vi "Match.vi"(10 "log record":T1 {"timestamp" format="%<%x %.3X>T"}, 11 "regex":refnum<class "Regex.lvclass">) -> (2 "matches":bool[](array[boolean]), 3 "dup regex":refnum<class "Regex.lvclass">)   [LabVIEW 2018, in "Logging.lvlib" / "Regex.lvclass"]
uses:
  Regex.lvclass
  Log Record.ctl
  Logger/Internal Log Levels.ctl
  Regex.lvclass/Regex.ctl
  <vilib>/regexp/Match Regular Expression.xnode
  Logging.lvlib
panel:
  # "Connector Pane"
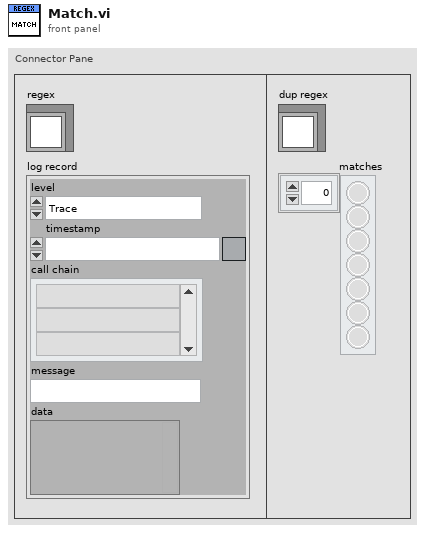
[diagram p1: front panel]
types:
  T1 = typedef "Logging.lvlib/Log Record.ctl" = cluster{"level":T2, "timestamp":timestamp, "call chain":string[], "message":string, "data":variant}
  T2 = typedef "Logging.lvlib/Internal Log Levels.ctl" = enum16{"Trace", "Debug", "Info", "Warning", "Error", "Critical", "Internal"}
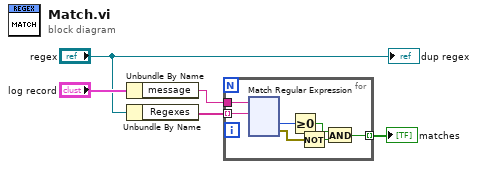
[diagram p0: block diagram]
diagram:
  n1 = Unbundle By Name("log record") -> ("message"=w4:string)
  n2 = Unbundle By Name("regex") -> ("Regexes"=w3:string[])
  n3 = for {
    tunnel: w4 -> [w12]
    tunnel: w3 -> [w11] mode=indexing
    tunnel: [w7] -> w1 mode=indexing
    n4 = xnode "Match Regular Expression"("input string"=w12, "regular expression"=w11) -> ("offset past match"=w10:i32, "error out"=w8:errorcluster)  [unwired: 4 in, 3 out]
    n5 = Greater Or Equal To 0?(x=w10) -> (x >= 0?=w9:bool)
    n6 = Not(x=w8) -> (.not. x?=w6:bool)
    n7 = And(x=w9, y=w6) -> (x .and. y?=w7:bool)
  }
  "matches" <- w1
  "dup regex" <- "regex"
